vi "ST5520_CMD_2.vi"(8 "errin":errorcluster caption="entrée d'erreur (pas d'erreur)", 10 "VISA":string) -> (0 "errout":errorcluster caption="sortie d'erreur", 1 "DATA FINAL FLT":dbl, 2 "DATAOUT":string, 3 "60s?":bool, 4 "read buffer":string)   [LabVIEW 2020]
uses:
  OP500/VG/VG_progressBar.vi
  <instrlib>/HIOKI BT356X Series/HIOKI BT356X Series.lvlib
panel:
  in  "Arrêter":bool
  out "DATA LIVE":string
  # "DATA OUT"
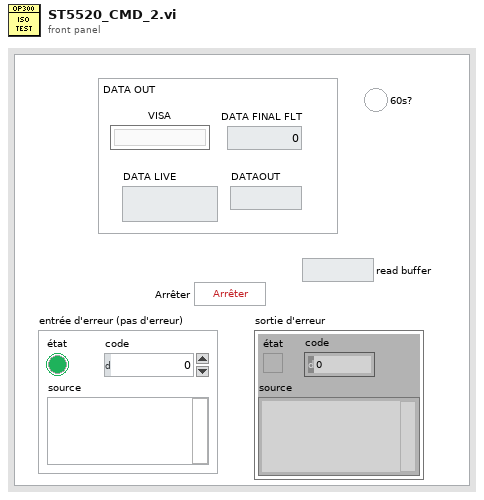
[diagram p1: front panel]
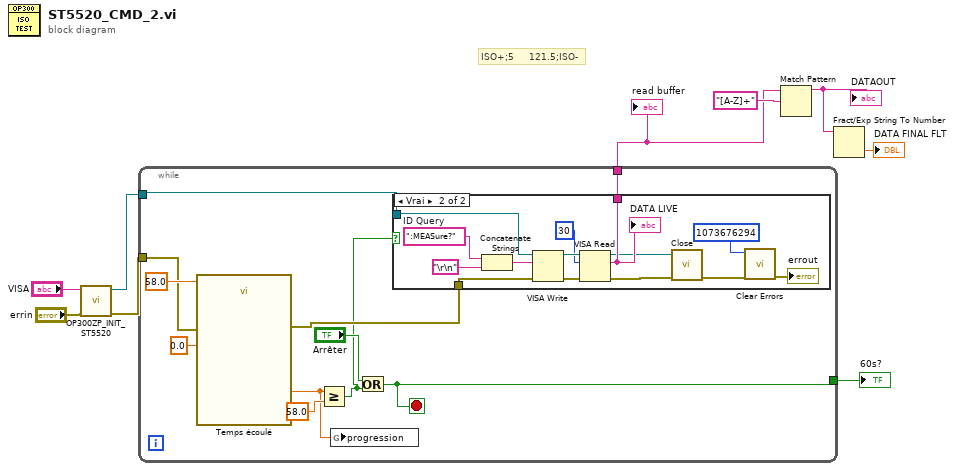
[diagram p0: block diagram]
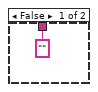
[diagram p2: hidden frame]
diagram:
  # "ISO+;5     121.5;ISO-"
  n1 = call "OP300ZP_INIT_ST5520.vi"("errin"="errin", "VISA"="VISA") -> ("errout"=w6:errorcluster, "VISA"=w7:refnum<visa-resource-name>)  [unwired: 8 in]
  n2 = while {
    tunnel: w6 -> [w14]
    tunnel: w7 -> [w20]
    tunnel: [w16] -> w2
    tunnel: [w15] -> w8
    stop <- w15 stop-if-true
    n3 = call "Temps écoulé"("Time Target (s)"=58.0, "error in (no error)"=w14, "Set Start Time (s)"=0.0) -> ("Elapsed Time (s)"=w11:dbl, "error out"=w12:errorcluster)  [unwired: 9 in, 6 out]
    n4 = Greater Or Equal?(x=w11, y=58.0) -> (x >= y?=w10:bool)
    n5 = global write "VG_progressBar.vi" "progression"(w11) -> ()
    n6 = Or(x="Arrêter", y=w10) -> (x .or. y?=w15:bool)
    n7 = case shown="Vrai" w10 {
      tunnel: w20 -> [_ w29]
      tunnel: ["" ("read buffer") w26] -> w16
      tunnel: w12 -> [_ w22]
      frame False {
      }
      frame True {
        w35 = ":MEASure?"  # ID Query
        n8 = Concatenate Strings(w35, "\r\n") -> (w31:string)
        n9 = VISA Write(VISA resource name=w29, write buffer=w31, error in (no error)=w22) -> (VISA resource name out=w34:refnum<visa-resource-name>, error out=w33:errorcluster)  [unwired: 1 out]
        n10 = VISA Read(VISA resource name=w34, byte count=u32 30 ("nombre d'octets"), error in (no error)=w33) -> (VISA resource name out=w23:refnum<visa-resource-name>, read buffer=w26:string, error out=w25:errorcluster)  [unwired: 1 out]
        "DATA LIVE" <- w26
        n11 = call <instrlib>:"Close.vi"("error in (no error)"=w25, "VISA resource name"=w23) -> ("error out"=w24:errorcluster)  [unwired: 9 in]
        n12 = call <vilib>:"Clear Errors.vi"("error in (no error)"=w24, "specific error code to clear (0: all)"=1073676294) -> ("error out"=→"errout":errorcluster)  [unwired: 4 in, 1 out]
      }
    }
  }
  "60s?" <- w8
  "read buffer" <- w2
  n13 = Match Pattern(string=w2, regular expression="[A-Z]+" ("expression régulière")) -> (before substring=w1:string)  [unwired: 1 in, 3 out]
  "DATAOUT" <- w1
  n14 = Fract/Exp String To Number(string=w1) -> (number=→"DATA FINAL FLT":dbl)  [unwired: 3 in, 1 out]
